vi "convert to packed lib type.vi"(8 "error in (no error)":errorcluster, 11 "PackedLibrary in":refnum<class "PackedLibrary.lvclass">) -> (0 "error out":errorcluster, 3 "NI_AB_API_PPL out":refnum<class "NI_AB_API_PPL.lvclass">)   [LabVIEW 2024, in "PackedLibrary.lvclass"]
uses:
  PackedLibrary.lvclass
  PackedLibrary.lvclass/PackedLibrary.ctl
  parent/Builder.lvclass
  <vilib>/AppBuilder/AB_API/PPL/NI_AB_API_PPL.lvclass
  D:/_repos/sandbox/github_p/labview-tools/cicd_tools/src/builders/parent/Builder.lvclass
  D:/_repos/sandbox/github_p/labview-tools/cicd_tools/src/builders/packed_library/PackedLibrary.lvclass
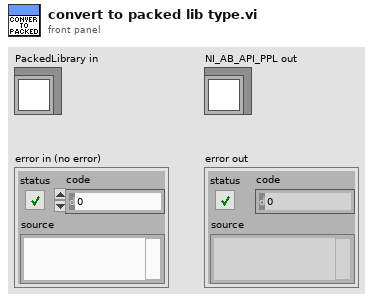
[diagram p1: front panel]
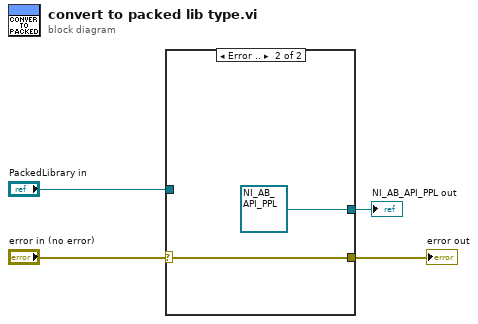
[diagram p0: block diagram]
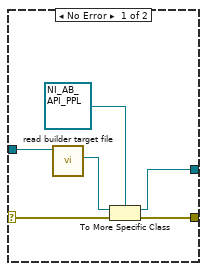
[diagram p2: hidden frame]
diagram:
  n1 = case shown="Error .." "error in (no error)" {
    selector: "error in (no error)" -> [w5 w12]
    tunnel: "PackedLibrary in" -> [w10 _]
    tunnel: [w9 refnum<class "NI_AB_API_PPL.lvclass"> refnum ("PPL out")] -> w3
    tunnel: [w6 w12] -> w2
    frame No Error {
      n2 = call "read builder target file.vi"("Builder in"=w10) -> ("builder target type"=w7:refnum<class "NI_AB_API_Build.lvclass">)  [unwired: 10 in]
      n3 = To More Specific Class(target class=refnum<class "NI_AB_API_PPL.lvclass"> refnum ("PPL out"), reference=w7, error in=w5) -> (specific class reference=w9:refnum<class "NI_AB_API_PPL.lvclass">, error out=w6:errorcluster)
    }
    frame Error {
    }
  }
  "NI_AB_API_PPL out" <- w3
  "error out" <- w2
